vi "Write Shape.vi"(8 "error in (no error)":errorcluster, 10 "Shape":T1, 11 "FSM.Node in":refnum<class "FSM.Node.lvclass">) -> (0 "error out":errorcluster, 3 "FSM.Node out":refnum<class "FSM.Node.lvclass">)   [LabVIEW 2020, in "FSM.Node.lvclass"]
uses:
  FSM.Node.lvclass
  Shape.ctl
  FSM.Node.lvclass/FSM.Node.ctl
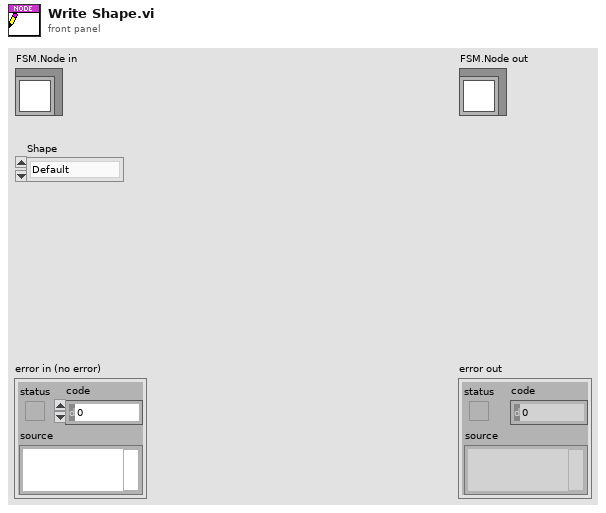
[diagram p1: front panel]
types:
  T1 = typedef "FSM.Node.lvclass/Shape.ctl" = enum16{"Default", "Start", "Action", "End"}
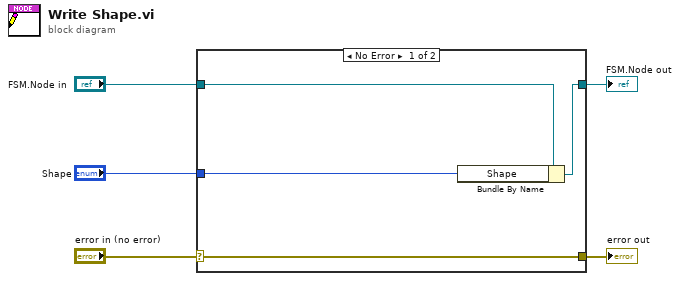
[diagram p0: block diagram]
diagram:
  n1 = case shown="No Error" "error in (no error)" {
    selector: "error in (no error)" -> [w9 w10]
    tunnel: [w9 w10] -> w4
    tunnel: [w7 w11] -> w2
    tunnel: "FSM.Node in" -> [w8 w11]
    tunnel: "Shape" -> [w6 _]
    frame No Error {
      n2 = Bundle By Name(cluster=w8, "Shape"=w6) -> (w7:refnum<class "FSM.Node.lvclass">)
    }
    frame Error {
    }
  }
  "error out" <- w4
  "FSM.Node out" <- w2
